vi "Get Ingredients.vi"(8 "error in (no error)":errorcluster, 11 "Plastic in":refnum<class "Plastic.lvclass">) -> (0 "error out":errorcluster, 2 "Ingredients":T1[](array[typedef]), 3 "Plastic out":refnum<class "Plastic.lvclass">)   [LabVIEW 2020, in "Plastic.lvclass"]
uses:
  Plastic.lvclass
  Item/Ingredient.ctl
  Item/Item.lvclass
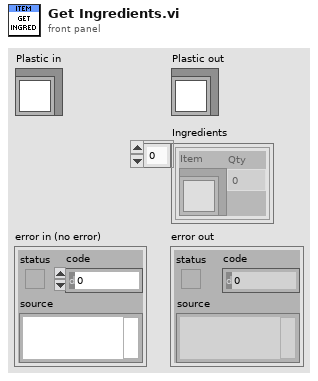
[diagram p1: front panel]
types:
  T1 = typedef "Item.lvclass/Ingredient.ctl" = cluster{"Item":refnum<class "Item.lvclass">, "Qty":dbl}
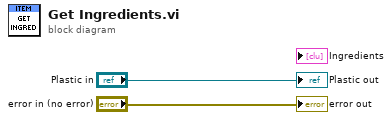
[diagram p0: block diagram]
diagram:
  "error out" <- "error in (no error)"
  "Plastic out" <- "Plastic in"
